vi "ExecutionView(CSM).vi"(7 "Name(\"\" to use uuid)":string="TestStandOI") -> ()   [LabVIEW 2020, in "CSMStand(Lite).lvlib"]
doc: "------------- lvcsm -------------\n[CSMStates]\nItem 0 = \"Idle\"\nItem 1 = \"CSM Documentation\"\nItem 2 = \"Error Handler\"\nItem 3 = \"VI Reference\"\nItem 4 = \"Critical Error\"\nItem 5 = \"Target Timeout Error\"\nItem 6 = \"Target Error\"\nItem 7 = \"Async Response\"\nItem 8 = \"Response\"\nItem 9 = \"Async Message Posted\"\nItem 10 = \"Initialize Core Data\"\nItem 11 = \"Exit\"\nItem 12 = \"Data: Initialize\"\nItem 13 = \"Data: Get Configuration\"\nItem 14 = \"Data: Get Internal Data\"\nItem 15 = \"Data: Set Configuration\"\nItem 16 = \"Data: Cleanup\"\nItem 17 = \"UI: Initialize\"\nItem 18 = \"UI: Cursor Set\"\nItem 19 = \"UI: Front Panel State\"\nItem 20 = \"Macro: Initialize\"\nItem 21 = \"Macro: Exit\"\nItem 22 = \"TS: Load Sequence\"\nItem 23 = \"TS: Test Started Handler\"\nItem 24 = \"TS: Step Start Handler\"\nItem 25 = \"TS: Step Complete Handler\"\nItem 26 = \"TS: Test Complete Handler\"\nItem 27 = \"Internal: action1\"\nItem 28 = \"Internal: action2\"\n\n[CSMStatus]\nItem 0 = \"Error Occurred@Error Handler\""
uses:
  CSMStand(Lite).lvlib
  <vilib>/Utility/miscctls.llb/LVRowAndColumnTypeDef.ctl
  Engine/Typedef/Def-StepComplete Event Data.ctl
  49887391-5aaa-4a15-bec5-64cc18cfe9d0.vi
  d29669de-e3bc-4aa1-abb6-bef5024a48d5.vi
  844f5a0a-3cc9-4d1a-ab8e-12611138b1fa.vi
  f99f0b71-739f-43a4-ba27-9b21da8a90fc.vi
  <userlib>/_NEVSTOP/Communicable State Machine(CSM)/_Support/Common/Format Timestamp.vi
  <userlib>/_NEVSTOP/Communicable State Machine(CSM)/AdvanceAPI/CSM - Make String Arguments Safe.vi
  <userlib>/_NEVSTOP/Communicable State Machine(CSM)/AdvanceAPI/CSM - Break Down Multiple States String.vi
  <userlib>/_NEVSTOP/Communicable State Machine(CSM)/AdvanceAPI/CSM - Compact Multiple States.vi
  <userlib>/_NEVSTOP/Communicable State Machine(CSM)/_Support/GlobalEvent/GEvt-Generate with Rule Check.vi
  <userlib>/_NEVSTOP/Communicable State Machine(CSM)/AdvanceAPI/CSM - Keywords.vi
  <userlib>/_NEVSTOP/Communicable State Machine(CSM)/_Shared/Trim Single-line Text.vi
  <userlib>/_NEVSTOP/Communicable State Machine(CSM)/_Support/GlobalEvent/Cache-GEvt Refs.vi
  <userlib>/_NEVSTOP/Communicable State Machine(CSM)/_Support/GlobalEvent/LogFilter/LogFilter - Check.vi
  <userlib>/_NEVSTOP/Communicable State Machine(CSM)/addons/API-String-Arugments-Support/_Support/Query Data as API String Arguments(variant).vi
  <userlib>/_NEVSTOP/Communicable State Machine(CSM)/addons/API-String-Arugments-Support/_Support/Convert API String Arguments to Data(variant).vi
  <userlib>/_NEVSTOP/Communicable State Machine(CSM)/_Support/GlobalEvent/LogFilter/LogFilter.lvclass
  <userlib>/_NEVSTOP/Communicable State Machine(CSM)/Communicable State Machine.lvlib
panel:
  in  "Sequence Viewer":i32(listbox)
  out "State History":string
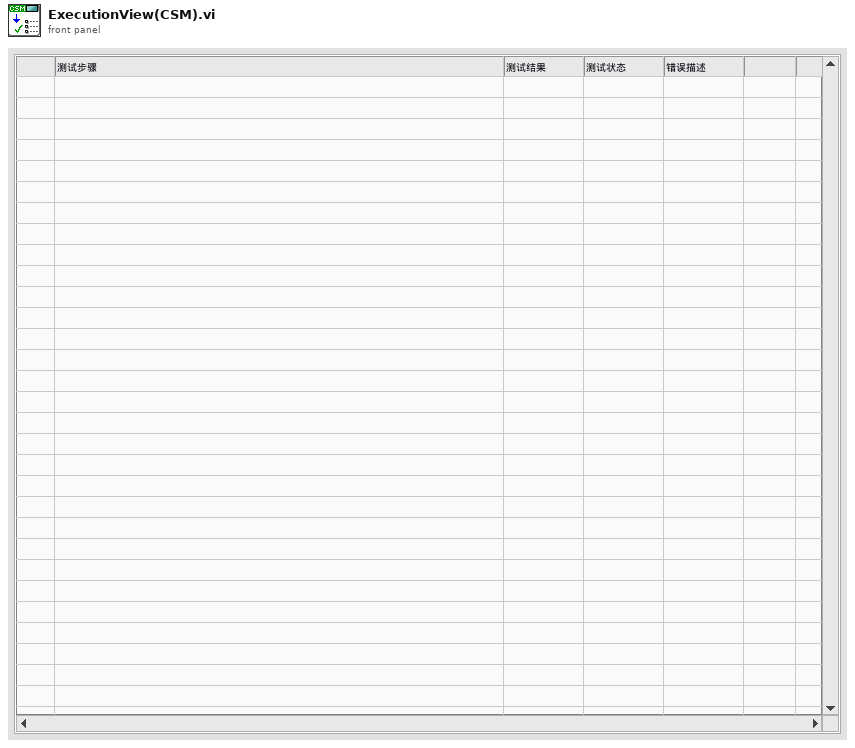
[diagram p1: front panel]
types:
  T1 = enum32{"Invalid", "Standard", "Closed", "Hidden", "Minimized", "Maximized"}
  T2 = enum32{"invalid app kind", "Development System", "Run Time System", "Student Edition", "Embedded LabVIEW", "Evaluation", "Custom"}
  T3 = typedef "LVRowAndColumnTypeDef.ctl" = cluster{"Row":i32, "Column":i32}
  T4 = typedef "CSMStand(Lite).lvlib/Def-StepComplete Event Data.ctl" = cluster{"index":i32, "Arguments":string, "error":errorcluster}
  T5 = typedef "Communicable State Machine.lvlib/_CSM_Response Source Message.ctl" = cluster{"‘State":string, "’Arguments":string, "’Error":errorcluster}
  T6 = cluster{"Current VI Reference":refnum<vi>, "Close Panel on Exit?":bool}
  T7 = cluster{"Core":cluster{"Current VI Reference":refnum<vi>, "Close Panel on Exit?":bool}, "Sequence Viewer":refnum<vi>, "ResponseMaxLen":i32}
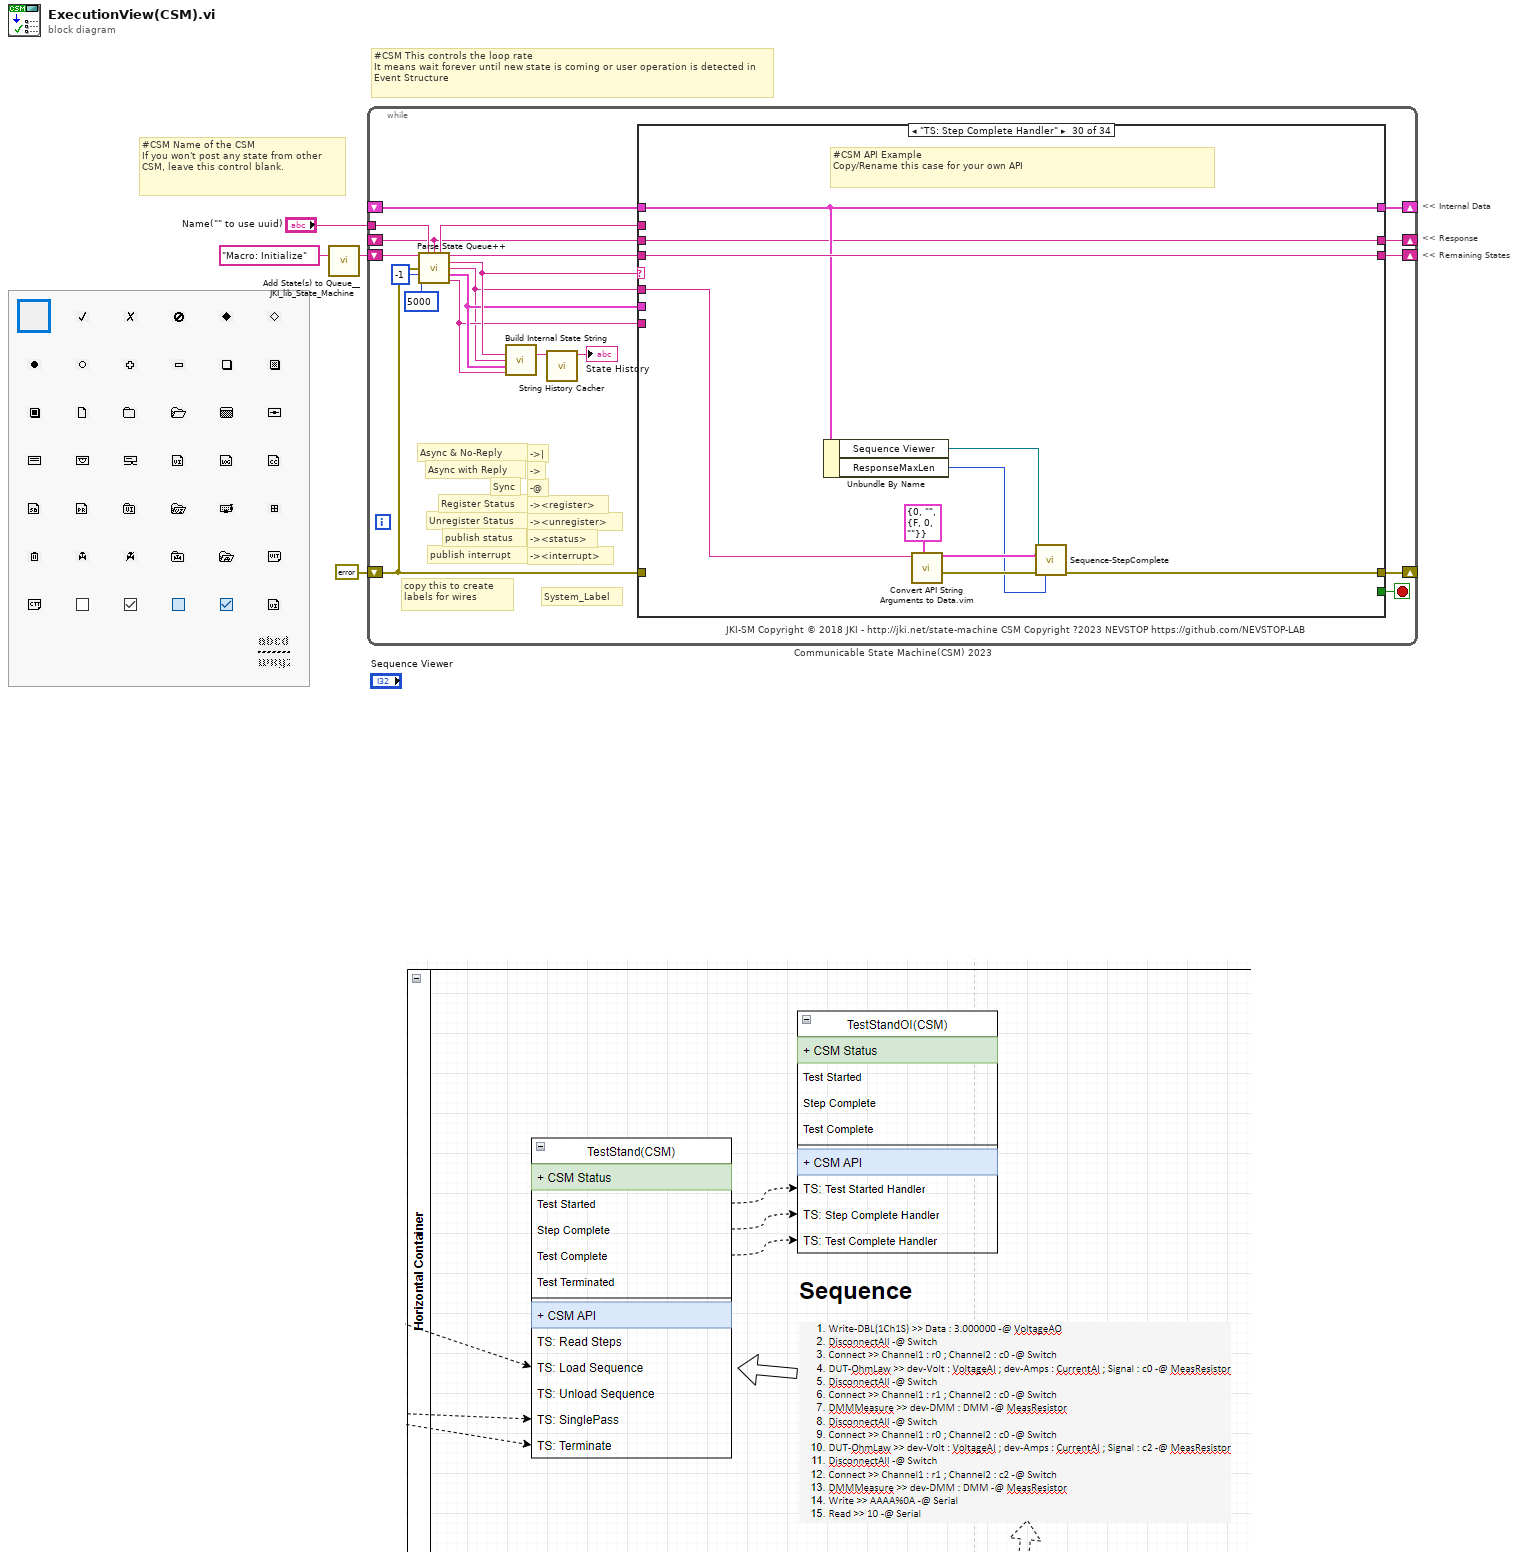
[diagram p0: block diagram]
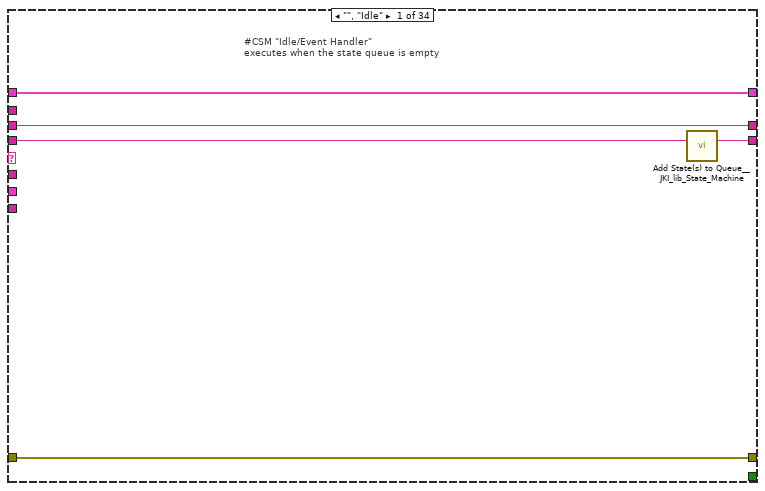
[diagram p2: hidden frame]
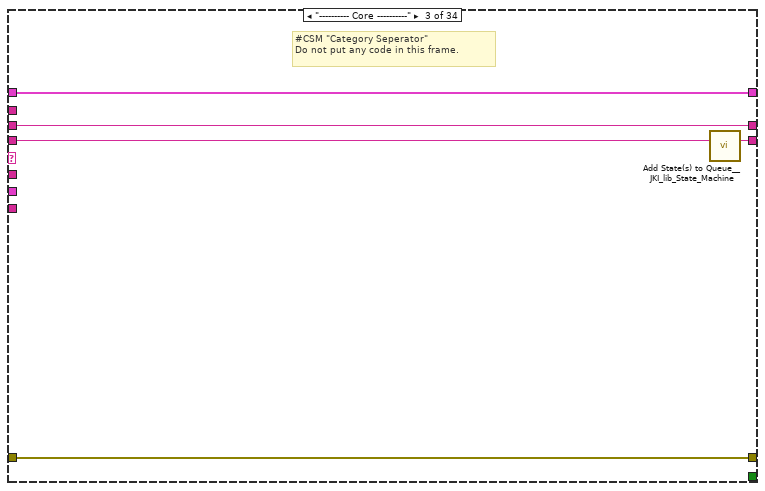
[diagram p4: hidden frame]
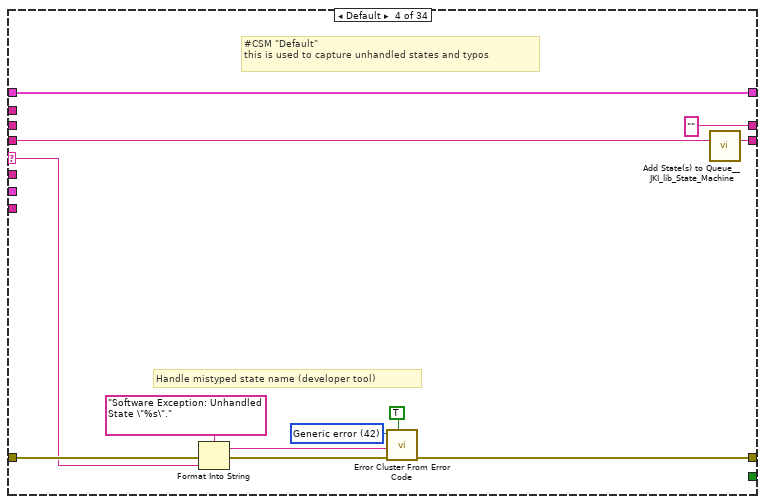
[diagram p5: hidden frame]
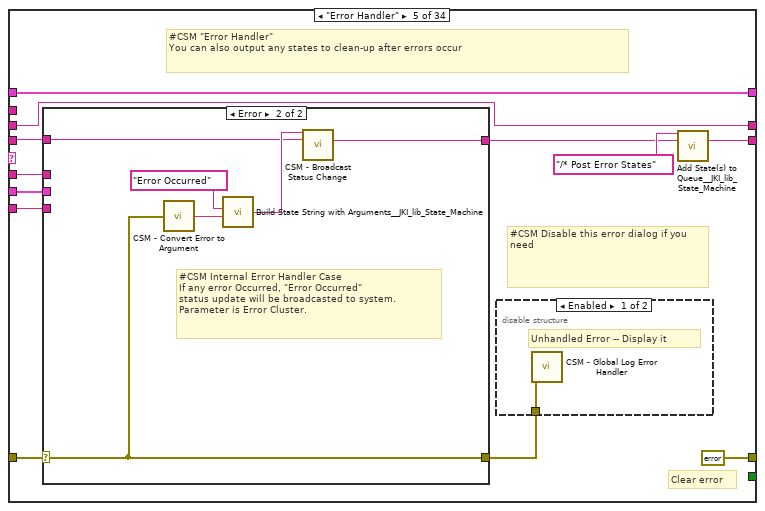
[diagram p6: hidden frame]
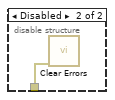
[diagram p7: hidden frame]
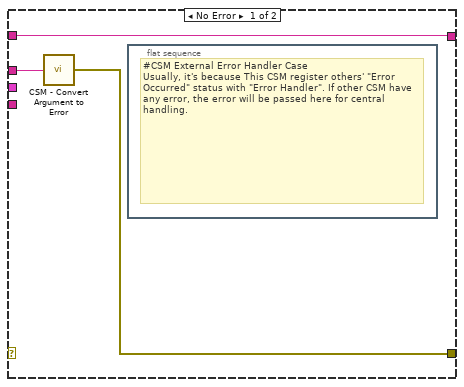
[diagram p8: hidden frame]
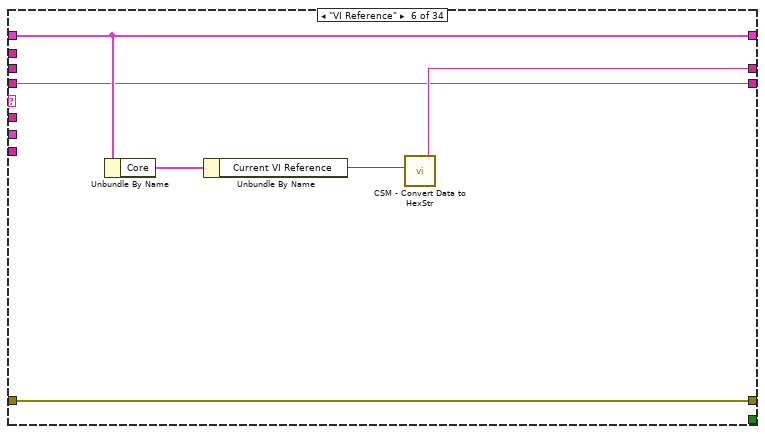
[diagram p9: hidden frame]
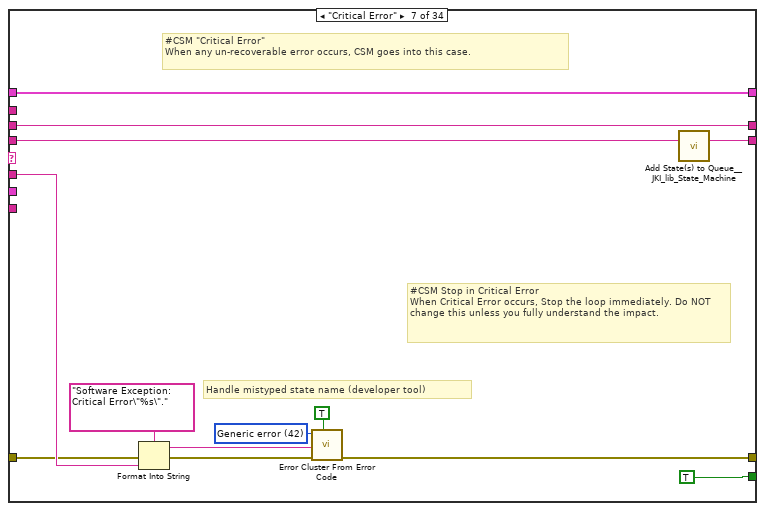
[diagram p10: hidden frame]
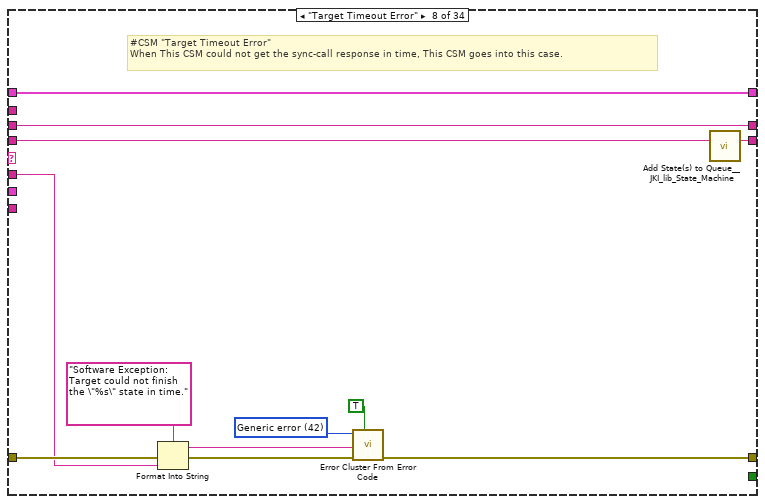
[diagram p11: hidden frame]
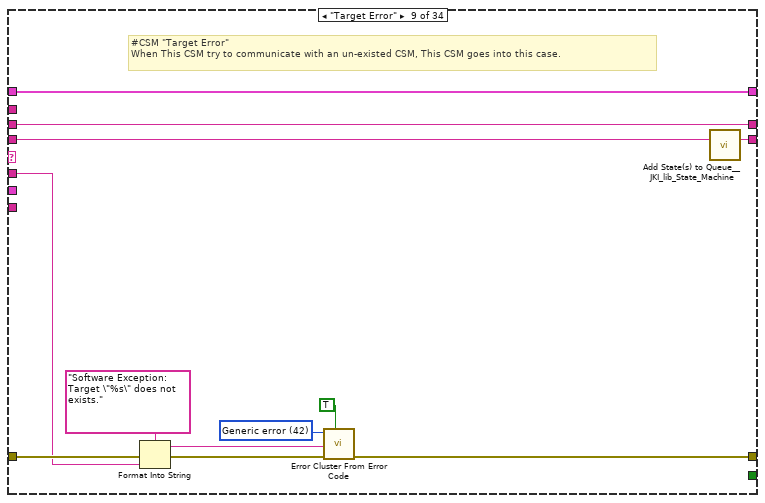
[diagram p12: hidden frame]
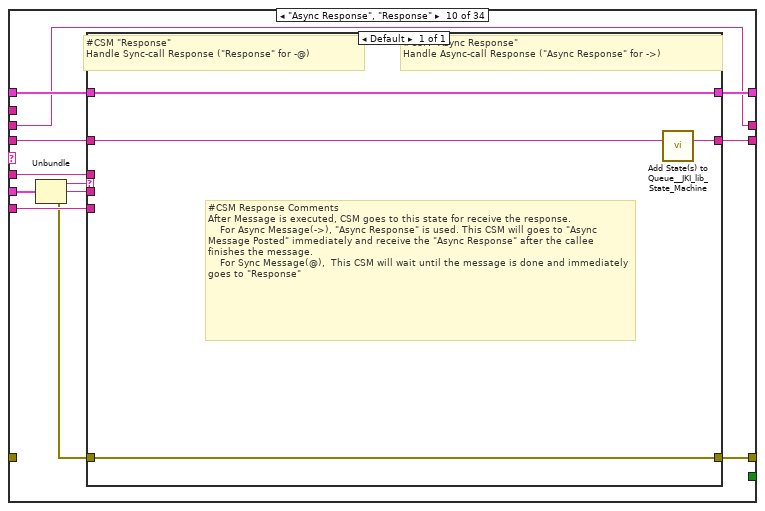
[diagram p13: hidden frame]
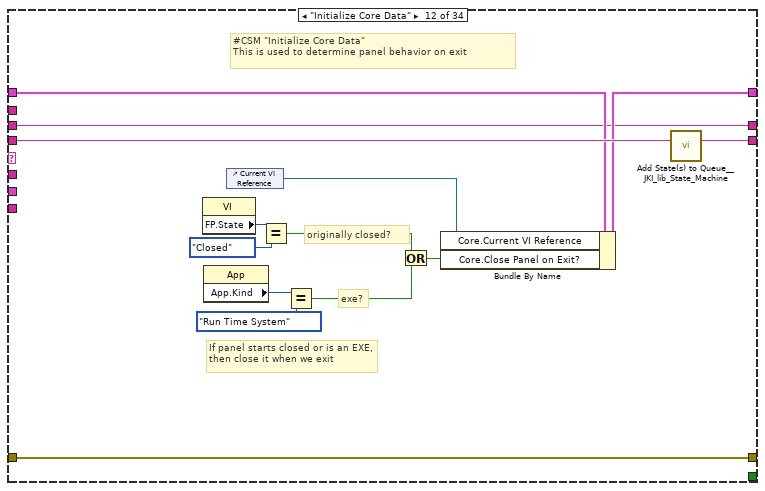
[diagram p15: hidden frame]
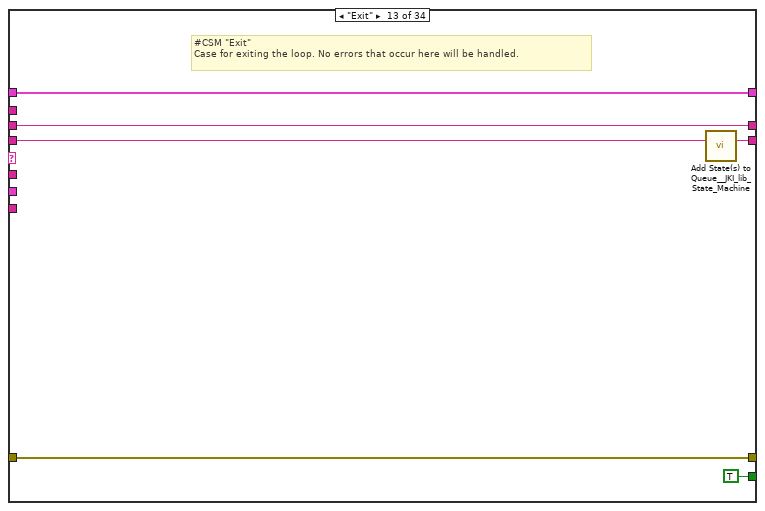
[diagram p16: hidden frame]
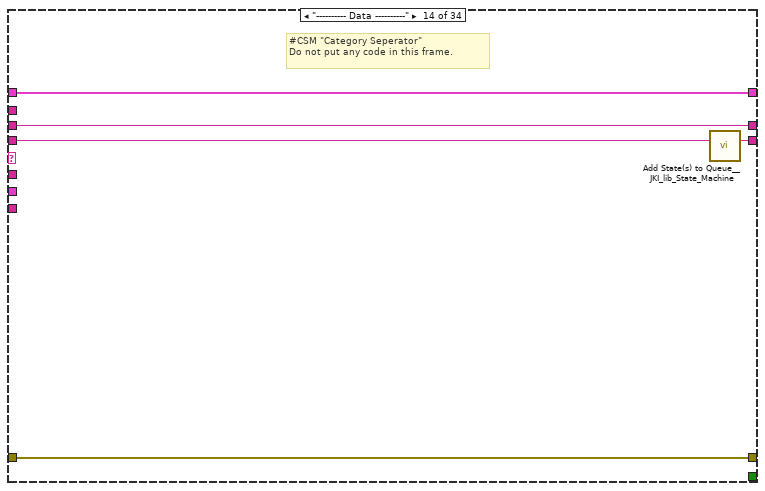
[diagram p17: hidden frame]
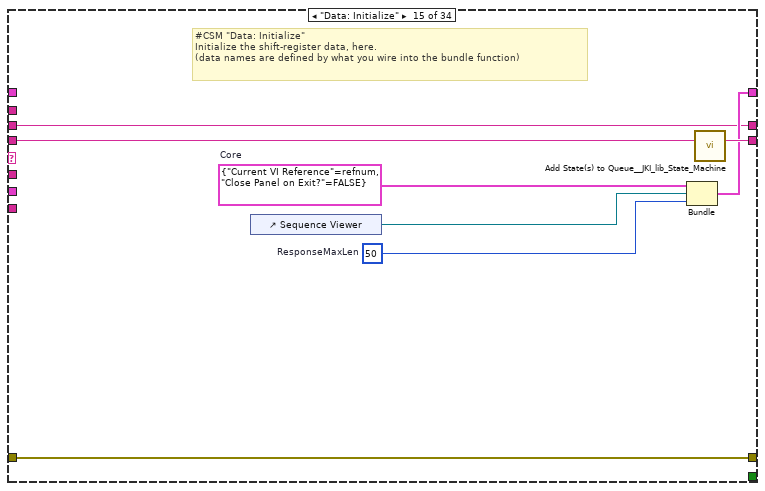
[diagram p18: hidden frame]
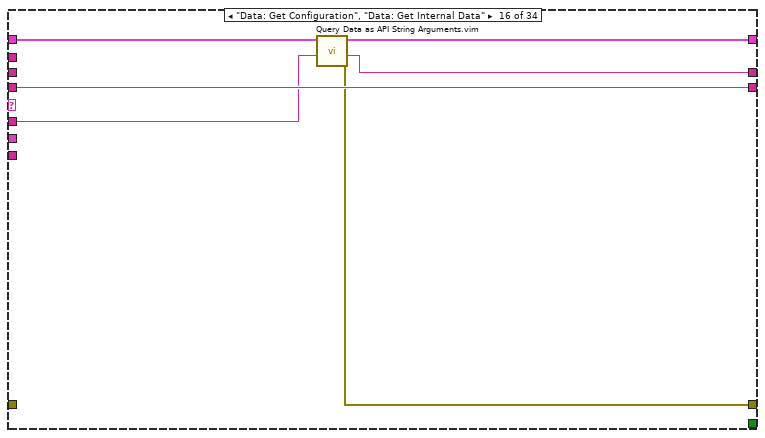
[diagram p19: hidden frame]
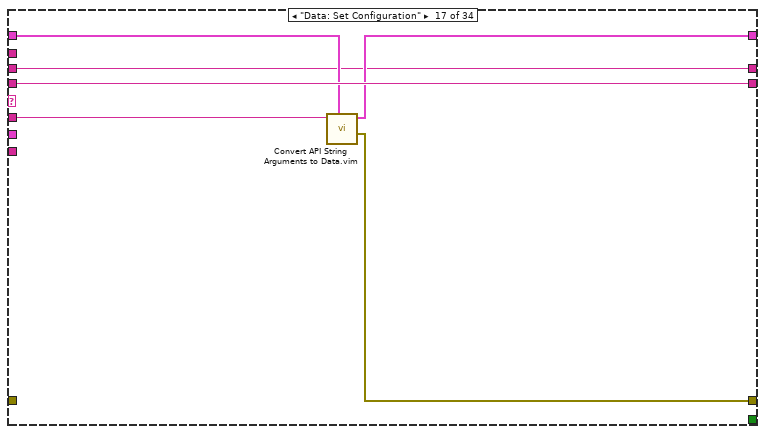
[diagram p20: hidden frame]
diagram:
  # "<< Internal Data"
  # "<< Response"
  # "<< Remaining States"
  # "#CSM Name of the CSM\nIf you won't post any state from other CSM, leave this control blank."
  # "#CSM This controls the loop rate\nIt means wait forever until new state is coming or user operation is detected in Event Structure"
  n1 = call <vilib>:"Add State(s) to Queue__JKI_lib_State_Machine.vi"("State(s) in (\"\")"="Macro: Initialize" ("Init State(\"Macro: Initialize\")")) -> ("States Out"=w1:string)  [unwired: 14 in]
  n2 = while "Communicable State Machine(CSM) 2023" {
    shift-right: [w19] -> _
    shift-left: _ -> [w18]
    shift-right: [w22] -> _
    shift-left: errorcluster {"status"=FALSE, "code"=0, "source"=""} ("error out") -> [w17]
    shift-right: [w21] -> _
    shift-left: w1 -> [w23]
    tunnel: "Name(\"\" to use uuid)" -> [w14]
    shift-right: [w15] -> _
    shift-left: _ -> [w7]
    stop <- w20 stop-if-true
    # "-><interrupt>"
    # "-><status>"
    # "-><unregister>"
    # "-><register>"
    # "-@"
    # "->"
    # "->|"
    # "publish interrupt"
    # "publish status"
    # "Unregister Status"
    # "Register Status"
    # "Sync"
    # "Async with Reply"
    # "Async & No-Reply"
    # "copy this to create labels for wires"
    # "System_Label"
    # "JKI-SM Copyright © 2018 JKI - http://jki.net/state-machine CSM Copyright ?2023 NEVSTOP https://github.com/NEVSTOP-LAB"
    n3 = call <userlib>:"Parse State Queue++.vi"("State Queue"=w23, "Name (\"\" to Use UUID)"=w14, "Response Arguments"=w7, "Previous Error"=w17, "Dequeue (1 ms)"=-1 ("Dequeue Timeout(0ms)"), "Response Timeout (-2 Use Global Settings)"=5000 ("Response Timeout(1000ms)")) -> ("Name Used"=w8:string, "Remaining States"=w24:string, "Current State"=w11:string, "Arguments"=w6:string, ">> Response Source Message >>"=w10:T5, ">> Source CSM >>"=w9:string)  [unwired: 4 in]
    n4 = call <userlib>:"Build Internal State String.vi"("State"=w11, "Arguments (\"\")"=w6, ">> Response Source Message >>"=w10, "Source (\"\")"=w9) -> ("State With Arguments"=w12:string)  [unwired: 11 in]
    n5 = call <userlib>:"String History Cacher.vi"("String"=w12) -> ("String Cache"=→"State History":string)  [unwired: 10 in]
    n6 = case shown="\"TS: Step Complete Handler\"" w11 {
      selector: w11 -> [_ _ _ w40 _ _ _ _ _ _ _ _ _ _ _ _ _ _ _ _ _ _ _ _ _ _ _ _ _ _ _ _ _ _]
      tunnel: w24 -> [w26 w33 w38 w44 w56 w75 w91 w99 w111 w127 w135 w150 w156 w161 w169 w175 w181 w188 w193 w215 w222 w238 w308 w314 w326 w329 w339 w346 w355 w365 w368 w374 w379 w384]
      tunnel: w6 -> [_ _ _ _ w54 _ w84 w95 w107 w121 _ _ _ _ _ w172 w180 _ _ _ w217 w232 _ _ _ _ w332 _ w349 w359 _ _ _ _]
      tunnel: w18 -> [w27 w32 w35 w42 w61 w79 w92 w97 w109 w125 w134 w143 w154 w158 _ w174 w179 w183 w190 w213 w220 w234 w305 w311 w323 w328 w337 w343 w354 w364 w367 w371 w376 w381]
      tunnel: [w28 w31 w36 w46 errorcluster {"status"=FALSE, "code"=0, "source"=""} ("error out") w74 w81 w94 w106 w124 w136 w147 w153 w159 w166 w170 w177 w184 w191 w197 w218 w235 w306 w312 w324 w330 w334 w341 w352 w362 w369 w372 w377 w382] -> w22
      tunnel: w17 -> [w28 w31 w36 w45 w60 w74 w82 w100 w112 _ w136 w147 w153 w159 w166 _ _ w185 w191 w210 w219 w236 w306 w312 w324 w330 w333 w344 _ _ w369 w372 w377 w382]
      tunnel: [w29 w33 w37 w43 w58 w75 w90 w98 w110 w128 w135 w149 w155 w160 w168 w175 w181 w187 w192 w214 w221 w237 w307 w313 w325 w329 w338 w345 w355 w365 w368 w373 w378 w383] -> w21
      tunnel: [_ _ _ _ _ _ TRUE _ _ _ _ _ TRUE _ _ _ _ _ _ _ _ _ _ _ _ _ _ _ _ _ _ _ _ _] -> w20
      tunnel: [w27 w32 w35 w42 w61 w79 w92 w97 w109 w126 w134 w148 w154 w158 w167 w173 w178 w183 w190 w213 w220 w234 w305 w311 w323 w328 w337 w343 w354 w364 w367 w371 w376 w381] -> w19
      tunnel: w9 -> [_ _ _ _ w53 _ _ _ _ w122 _ _ _ _ _ _ _ _ _ _ _ _ _ _ _ _ _ _ _ _ _ _ _ _]
      tunnel: w10 -> [_ _ _ _ w52 _ _ _ _ w123 _ _ _ _ _ _ _ _ _ _ _ _ _ _ _ _ _ _ _ _ _ _ _ _]
      tunnel: [w25 w30 w34 "" w51 w76 w80 w93 w105 w117 w133 w137 w151 w157 w163 w171 w176 w182 w189 w194 w216 w231 w304 w309 w315 w327 w331 w340 w347 w357 w366 w370 w375 w380] -> w15
      tunnel: w8 -> [_ _ _ _ _ _ _ _ _ _ _ _ _ _ _ _ _ _ _ _ _ _ _ _ _ _ _ _ _ _ _ _ _ _]
      tunnel: w7 -> [w25 w30 w34 _ w51 _ w80 w93 w105 w117 w133 w137 w151 w157 w163 _ w176 w182 w189 w194 w216 w231 w304 w309 w315 w327 w331 w340 w347 w357 w366 w370 w375 w380]
      frame "", "Idle" {
        # "#CSM \"Idle/Event Handler\"\nexecutes when the state queue is empty"
        n7 = call <vilib>:"Add State(s) to Queue__JKI_lib_State_Machine.vi"("State(s) in (\"\")"=w26) -> ("States Out"=w29:string)  [unwired: 14 in]
      }
      frame "CSM Documentation" {
        # "CSM Documentation"
        # "#CSM State Syntax\n\n// Comment line, all text to the right of “//” will be ignored\n// Local Message Example\nDoSth: DoA >> Arguments\n\n// Sync Call Example\nAPI: xxxx >> Arguments -@ TargetModule\n\n// Async Call Example\nAPI: xxxx >> Arguments -> TargetModule\n\n// Async Call without Reply Example\nAPI: xxxx >> Arguments ->| TargetModule\n\n// Broadcast normal status:\nStatus >> StatusArguments  -><status>\n\n// Broadcast Interrupt status:\nInterrupt >> StatusArguments  -><interrupt>\n\n// Register Source Module's status to Handler Module\nStatus@Source Module >> Handler Module@Handler Module -><register>\n\n// Unegister Source Module's status\nStatus@Source Module >> Handler Module -><unregister>"
        # "#CSM README FIRST\n\nCSM is a LabVIEW application framework that builds upon JKI State Machine (JKISM). It follows the pattern of JKISM and extends the keywords to describe message communication between CSM modules, including concepts such as Sync-Message, Async-Message, Subscription/Unsubscription of status - essential elements for creating reusable code modules. \n\nFor more information, please visit the CSM wiki: https://github.com/NEVSTOP-LAB/JKI-State-Machine-Plus-Plus/wiki\n\nFor instructions on JKI State Machine, visit: \n    http://jki.net/state-machine/\nFor information about CSM, visit: \n    https://github.com/NEVSTOP-LAB"
        # "#CSM \"Documentation\"\nCase for holding CSM Documenation"
      }
      frame "---------- Core ----------" {
        # "#CSM \"Category Seperator\"\nDo not put any code in this frame."
        n8 = call <vilib>:"Add State(s) to Queue__JKI_lib_State_Machine.vi"("State(s) in (\"\")"=w38) -> ("States Out"=w37:string)  [unwired: 14 in]
      }
      frame Default {
        w49 = 42 items=["No error", "Argument error", "Memory is full", "Out of zone", "End of file", "File already open", "Generic file I/O error", "File not found", "File permission error", "Disk is full", "Duplicate path", "Too many files open", "System feature not enabled", "Resource file not found", "Cannot add resource", "Resource not found", "Image not found", "Image memory error", "Pen does not exist", "Config type invalid", "Config token not found", "Config parse error", "Config memory error", "Bad external code format", "Bad external code offset", "External code not present", "Null window", "Destroy window error", "Null menu", "Print aborted", "Bad print record", "Print driver error", "Windows error during printing", "Memory error during printing", "Print dialog error", "Generic print error", "Invalid device refnum", "Device not found", "Device parameter error", "Device unit error", "Cannot open device", "Device call aborted", "Generic error", "Cancelled by user", "Object ID too low", "Object ID too high", "Object not in heap", "Unknown heap", "Unknown object (invalid DefProc)", "Unknown object (DefProc not in table)", "Message out of range", "Invalid (null) method", "Unknown message", "Manager call not supported", "Bad address", "Network operation in progress", "Network operation timed out", "Connection is busy", "Network attribute not supported", "Network error", "Address in use", "System out of memory", "Connection aborted", "Connection refused", "Not connected", "Already connected", "Connection closed", "Initialization error (interapplication manager)", "Bad occurrence", "Wait on unbound occurrence handler", "Occurrence queue overflow", "Datalog type conflict", "Unused", "Unrecognized type (interapplication manager)", "Memory corrupt", "Failed to make temporary DLL", "Old CIN version", "Drag socket not found", "Failed to load drop-object", "Failed to register OLE object", "Failed to release OLE object", "Format specifier type mismatch", "Unknown format specifier", "Too few format specifiers", "Too many format specifiers", "Scan failed", "Newer CIN version", "Error converting to variant", "Runtime menu error", "Password tampered", "Variant attribute not found", "Incompatible variant data type", "Event data is not available", "Event Store is not present", "Occurrence is not found", "Event Queue is not created", "Event info is not available", "Refnum passed is NULL", "Error retrieving Class GUID", "Error retrieving CoClass GUID", "Error retrieving TypeLib GUID.", "Bad built application magic bytes.", "Specific driver is different from the specific driver associated with the Logical Name.", "There is no session opened to the class driver.", "Max Error", "MAX - Error with config objects", "MAX - Error loading configuration", "MAX - Group not supported"]
        # "#CSM \"Default\"\nthis is used to capture unhandled states and typos"
        # "Handle mistyped state name (developer tool)"
        n9 = Format Into String(format string="Software Exception: Unhandled State \"%s\"." ("message"), error in=w45, w40) -> (resulting string=w48:string, error out=w47:errorcluster)  [unwired: 1 in]
        n10 = call <vilib>:"Error Cluster From Error Code.vi"("show call chain? (False)"=TRUE, "error in (no error)"=w47, "error message (\"\")"=w48, "error code (0)"=w49) -> ("error out"=w46:errorcluster)  [unwired: 5 in]
        n11 = call <vilib>:"Add State(s) to Queue__JKI_lib_State_Machine.vi"("State(s) in (\"\")"=w44) -> ("States Out"=w43:string)  [unwired: 14 in]
      }
      frame "Error Handler" {
        # "#CSM Disable this error dialog if you need"
        # "#CSM \"Error Handler\"\nYou can also output any states to clean-up after errors occur"
        # "Clear error"
        n12 = case shown="Error" w60 {
          selector: w60 -> [_ w68]
          tunnel: [w66 w70] -> w57
          tunnel: w56 -> [w66 w69]
          tunnel: [w65 w68] -> w55
          tunnel: w54 -> [w67 _]
          tunnel: w53 -> [_ _]
          tunnel: w52 -> [_ _]
          frame No Error {
            n13 = call <userlib>:"CSM - Convert Argument to Error.vi"("Argument"=w67) -> ("Error"=w65:errorcluster)  [unwired: 4 in]
            n14 = flat-sequence {
              frame #0 {
                # "#CSM External Error Handler Case\nUsually, it's because This CSM register others' \"Error Occurred\" status with \"Error Handler\". If other CSM have any error, the error will be passed here for central handling."
              }
            }
          }
          frame Error {
            # "#CSM Internal Error Handler Case \nIf any error Occurred, \"Error Occurred\" \nstatus update will be broadcasted to system.\nParameter is Error Cluster."
            n15 = call <userlib>:"CSM - Convert Error to Argument.vi"("Error"=w68) -> ("Argument"=w72:string)  [unwired: 4 in]
            n16 = call <vilib>:"Build State String with Arguments__JKI_lib_State_Machine.vi"("Arguments (\"\")"=w72, "State"="Error Occurred" ("Status with Arguments")) -> ("State with Arguments"=w71:string)  [unwired: 4 in]
            n17 = call <userlib>:"CSM - Broadcast Status Change.vi"("Status With Arguments"=w71, "State Queue"=w69) -> ("Remaining States"=w70:string)  [unwired: 13 in]
          }
        }
        n18 = disable-structure shown="Enabled" {
          disable-tunnel: w55 -> [w63 w64]
          frame Enabled {
            # "Unhandled Error -- Display it"
            n19 = call <userlib>:"CSM - Global Log Error Handler.vi"("Error In"=w63) -> ()  [unwired: 10 in, 1 out]
          }
          frame Disabled {
            n20 = call <vilib>:"Clear Errors.vi"("error in (no error)"=w64) -> ()  [unwired: 5 in, 2 out]
          }
        }
        n21 = call <vilib>:"Add State(s) to Queue__JKI_lib_State_Machine.vi"("State(s) in Front (\"\")"="/* Post Error States", "State(s) in (\"\")"=w57) -> ("States Out"=w58:string)  [unwired: 13 in]
      }
      frame "VI Reference" {
        n22 = Unbundle By Name(w79) -> ("Core"=w78:T6)
        n23 = Unbundle By Name(w78) -> ("Current VI Reference"=w77:refnum<vi>)
        n24 = call <userlib>:"CSM - Convert Data to HexStr.vi"("Variant"=w77) -> ("HEX String (0-9,A-F)"=w76:string)  [unwired: 8 in]
      }
      frame "Critical Error" {
        w88 = 42 items=["No error", "Argument error", "Memory is full", "Out of zone", "End of file", "File already open", "Generic file I/O error", "File not found", "File permission error", "Disk is full", "Duplicate path", "Too many files open", "System feature not enabled", "Resource file not found", "Cannot add resource", "Resource not found", "Image not found", "Image memory error", "Pen does not exist", "Config type invalid", "Config token not found", "Config parse error", "Config memory error", "Bad external code format", "Bad external code offset", "External code not present", "Null window", "Destroy window error", "Null menu", "Print aborted", "Bad print record", "Print driver error", "Windows error during printing", "Memory error during printing", "Print dialog error", "Generic print error", "Invalid device refnum", "Device not found", "Device parameter error", "Device unit error", "Cannot open device", "Device call aborted", "Generic error", "Cancelled by user", "Object ID too low", "Object ID too high", "Object not in heap", "Unknown heap", "Unknown object (invalid DefProc)", "Unknown object (DefProc not in table)", "Message out of range", "Invalid (null) method", "Unknown message", "Manager call not supported", "Bad address", "Network operation in progress", "Network operation timed out", "Connection is busy", "Network attribute not supported", "Network error", "Address in use", "System out of memory", "Connection aborted", "Connection refused", "Not connected", "Already connected", "Connection closed", "Initialization error (interapplication manager)", "Bad occurrence", "Wait on unbound occurrence handler", "Occurrence queue overflow", "Datalog type conflict", "Unused", "Unrecognized type (interapplication manager)", "Memory corrupt", "Failed to make temporary DLL", "Old CIN version", "Drag socket not found", "Failed to load drop-object", "Failed to register OLE object", "Failed to release OLE object", "Format specifier type mismatch", "Unknown format specifier", "Too few format specifiers", "Too many format specifiers", "Scan failed", "Newer CIN version", "Error converting to variant", "Runtime menu error", "Password tampered", "Variant attribute not found", "Incompatible variant data type", "Event data is not available", "Event Store is not present", "Occurrence is not found", "Event Queue is not created", "Event info is not available", "Refnum passed is NULL", "Error retrieving Class GUID", "Error retrieving CoClass GUID", "Error retrieving TypeLib GUID.", "Bad built application magic bytes.", "Specific driver is different from the specific driver associated with the Logical Name.", "There is no session opened to the class driver.", "Max Error", "MAX - Error with config objects", "MAX - Error loading configuration", "MAX - Group not supported"]
        # "#CSM \"Critical Error\"\nWhen any un-recoverable error occurs, CSM goes into this case."
        # "#CSM Stop in Critical Error\nWhen Critical Error occurs, Stop the loop immediately. Do NOT change this unless you fully understand the impact."
        # "Handle mistyped state name (developer tool)"
        n25 = Format Into String(format string="Software Exception: Critical Error\"%s\"." ("message"), error in=w82, w84) -> (resulting string=w87:string, error out=w86:errorcluster)  [unwired: 1 in]
        n26 = call <vilib>:"Error Cluster From Error Code.vi"("show call chain? (False)"=TRUE, "error in (no error)"=w86, "error message (\"\")"=w87, "error code (0)"=w88) -> ("error out"=w81:errorcluster)  [unwired: 5 in]
        n27 = call <vilib>:"Add State(s) to Queue__JKI_lib_State_Machine.vi"("State(s) in (\"\")"=w91) -> ("States Out"=w90:string)  [unwired: 14 in]
      }
      frame "Target Timeout Error" {
        w103 = 42 items=["No error", "Argument error", "Memory is full", "Out of zone", "End of file", "File already open", "Generic file I/O error", "File not found", "File permission error", "Disk is full", "Duplicate path", "Too many files open", "System feature not enabled", "Resource file not found", "Cannot add resource", "Resource not found", "Image not found", "Image memory error", "Pen does not exist", "Config type invalid", "Config token not found", "Config parse error", "Config memory error", "Bad external code format", "Bad external code offset", "External code not present", "Null window", "Destroy window error", "Null menu", "Print aborted", "Bad print record", "Print driver error", "Windows error during printing", "Memory error during printing", "Print dialog error", "Generic print error", "Invalid device refnum", "Device not found", "Device parameter error", "Device unit error", "Cannot open device", "Device call aborted", "Generic error", "Cancelled by user", "Object ID too low", "Object ID too high", "Object not in heap", "Unknown heap", "Unknown object (invalid DefProc)", "Unknown object (DefProc not in table)", "Message out of range", "Invalid (null) method", "Unknown message", "Manager call not supported", "Bad address", "Network operation in progress", "Network operation timed out", "Connection is busy", "Network attribute not supported", "Network error", "Address in use", "System out of memory", "Connection aborted", "Connection refused", "Not connected", "Already connected", "Connection closed", "Initialization error (interapplication manager)", "Bad occurrence", "Wait on unbound occurrence handler", "Occurrence queue overflow", "Datalog type conflict", "Unused", "Unrecognized type (interapplication manager)", "Memory corrupt", "Failed to make temporary DLL", "Old CIN version", "Drag socket not found", "Failed to load drop-object", "Failed to register OLE object", "Failed to release OLE object", "Format specifier type mismatch", "Unknown format specifier", "Too few format specifiers", "Too many format specifiers", "Scan failed", "Newer CIN version", "Error converting to variant", "Runtime menu error", "Password tampered", "Variant attribute not found", "Incompatible variant data type", "Event data is not available", "Event Store is not present", "Occurrence is not found", "Event Queue is not created", "Event info is not available", "Refnum passed is NULL", "Error retrieving Class GUID", "Error retrieving CoClass GUID", "Error retrieving TypeLib GUID.", "Bad built application magic bytes.", "Specific driver is different from the specific driver associated with the Logical Name.", "There is no session opened to the class driver.", "Max Error", "MAX - Error with config objects", "MAX - Error loading configuration", "MAX - Group not supported"]
        # "#CSM \"Target Timeout Error\"\nWhen This CSM could not get the sync-call response in time, This CSM goes into this case."
        n28 = Format Into String(format string="Software Exception: Target could not finish the \"%s\" state in time." ("message"), error in=w100, w95) -> (resulting string=w102:string, error out=w101:errorcluster)  [unwired: 1 in]
        n29 = call <vilib>:"Error Cluster From Error Code.vi"("show call chain? (False)"=TRUE, "error in (no error)"=w101, "error message (\"\")"=w102, "error code (0)"=w103) -> ("error out"=w94:errorcluster)  [unwired: 5 in]
        n30 = call <vilib>:"Add State(s) to Queue__JKI_lib_State_Machine.vi"("State(s) in (\"\")"=w99) -> ("States Out"=w98:string)  [unwired: 14 in]
      }
      frame "Target Error" {
        w115 = 42 items=["No error", "Argument error", "Memory is full", "Out of zone", "End of file", "File already open", "Generic file I/O error", "File not found", "File permission error", "Disk is full", "Duplicate path", "Too many files open", "System feature not enabled", "Resource file not found", "Cannot add resource", "Resource not found", "Image not found", "Image memory error", "Pen does not exist", "Config type invalid", "Config token not found", "Config parse error", "Config memory error", "Bad external code format", "Bad external code offset", "External code not present", "Null window", "Destroy window error", "Null menu", "Print aborted", "Bad print record", "Print driver error", "Windows error during printing", "Memory error during printing", "Print dialog error", "Generic print error", "Invalid device refnum", "Device not found", "Device parameter error", "Device unit error", "Cannot open device", "Device call aborted", "Generic error", "Cancelled by user", "Object ID too low", "Object ID too high", "Object not in heap", "Unknown heap", "Unknown object (invalid DefProc)", "Unknown object (DefProc not in table)", "Message out of range", "Invalid (null) method", "Unknown message", "Manager call not supported", "Bad address", "Network operation in progress", "Network operation timed out", "Connection is busy", "Network attribute not supported", "Network error", "Address in use", "System out of memory", "Connection aborted", "Connection refused", "Not connected", "Already connected", "Connection closed", "Initialization error (interapplication manager)", "Bad occurrence", "Wait on unbound occurrence handler", "Occurrence queue overflow", "Datalog type conflict", "Unused", "Unrecognized type (interapplication manager)", "Memory corrupt", "Failed to make temporary DLL", "Old CIN version", "Drag socket not found", "Failed to load drop-object", "Failed to register OLE object", "Failed to release OLE object", "Format specifier type mismatch", "Unknown format specifier", "Too few format specifiers", "Too many format specifiers", "Scan failed", "Newer CIN version", "Error converting to variant", "Runtime menu error", "Password tampered", "Variant attribute not found", "Incompatible variant data type", "Event data is not available", "Event Store is not present", "Occurrence is not found", "Event Queue is not created", "Event info is not available", "Refnum passed is NULL", "Error retrieving Class GUID", "Error retrieving CoClass GUID", "Error retrieving TypeLib GUID.", "Bad built application magic bytes.", "Specific driver is different from the specific driver associated with the Logical Name.", "There is no session opened to the class driver.", "Max Error", "MAX - Error with config objects", "MAX - Error loading configuration", "MAX - Group not supported"]
        # "#CSM \"Target Error\"\nWhen This CSM try to communicate with an un-existed CSM, This CSM goes into this case."
        n31 = Format Into String(format string="Software Exception: Target \"%s\" does not exists." ("message"), error in=w112, w107) -> (resulting string=w114:string, error out=w113:errorcluster)  [unwired: 1 in]
        n32 = call <vilib>:"Error Cluster From Error Code.vi"("show call chain? (False)"=TRUE, "error in (no error)"=w113, "error message (\"\")"=w114, "error code (0)"=w115) -> ("error out"=w106:errorcluster)  [unwired: 5 in]
        n33 = call <vilib>:"Add State(s) to Queue__JKI_lib_State_Machine.vi"("State(s) in (\"\")"=w111) -> ("States Out"=w110:string)  [unwired: 14 in]
      }
      frame "Async Response", "Response" {
        # "#CSM \"Async Response\"\nHandle Async-call Response (\"Async Response\" for ->)"
        # "#CSM \"Response\"\nHandle Sync-call Response (\"Response\" for -@)"
        n34 = Unbundle(w123) -> ("‘State"=w120:string, "’Arguments"=w119:string, "’Error"=w118:errorcluster)
        n35 = case shown="Default" w120 {
          tunnel: [w129] -> w128
          tunnel: w127 -> [w130]
          tunnel: [w132] -> w126
          tunnel: w125 -> [w132]
          tunnel: [w131] -> w124
          tunnel: w118 -> [w131]
          tunnel: w122 -> [_]
          tunnel: w121 -> [_]
          tunnel: w119 -> [_]
          frame Default {
            # "#CSM Response Comments\nAfter Message is executed, CSM goes to this state for receive the response.\n    For Async Message(->), \"Async Response\" is used. This CSM will goes to \"Async Message Posted\" immediately and receive the \"Async Response\" after the callee finishes the message.\n    For Sync Message(@),  This CSM will wait until the message is done and immediately goes to \"Response\""
            n36 = call <vilib>:"Add State(s) to Queue__JKI_lib_State_Machine.vi"("State(s) in (\"\")"=w130) -> ("States Out"=w129:string)  [unwired: 14 in]
          }
        }
      }
      frame "Async Message Posted" {
        # "#CSM \"Async Message Posted\"\nAfter Async Message is posted (-> or ->| ), CSM goes to this state for post-action.\nYou can use Argument - State to tell which Async Message is called."
      }
      frame "Initialize Core Data" {
        # "#CSM \"Initialize Core Data\"\nThis is used to determine panel behavior on exit"
        # "originally closed?"
        # "exe?"
        # "If panel starts closed or is an EXE, then close it when we exit"
        n37 = property class="VI"() -> ("FP.State"=w140:T1)  [unwired: 2 in, 2 out]
        n38 = property class="App"() -> ("App.Kind"=w146:T2)  [unwired: 2 in, 2 out]
        n39 = control-ref of="Current VI Reference"() -> (w141:refnum<vi>)
        n40 = Equal?(x=w140, y=T1."Closed" ("Front Panel Window:State")) -> (x = y?=w138:bool)
        n41 = Equal?(x=w146, y=T2."Run Time System" ("Application:Kind")) -> (x = y?=w144:bool)
        n42 = Or(x=w138, y=w144) -> (x .or. y?=w142:bool)
        n43 = Bundle By Name(cluster=w143, "Core.Current VI Reference"=w141, "Core.Close Panel on Exit?"=w142) -> (w148:T7)
        n44 = call <vilib>:"Add State(s) to Queue__JKI_lib_State_Machine.vi"("State(s) in (\"\")"=w150) -> ("States Out"=w149:string)  [unwired: 14 in]
      }
      frame "Exit" {
        # "#CSM \"Exit\"\nCase for exiting the loop. No errors that occur here will be handled."
        n45 = call <vilib>:"Add State(s) to Queue__JKI_lib_State_Machine.vi"("State(s) in (\"\")"=w156) -> ("States Out"=w155:string)  [unwired: 14 in]
      }
      frame "---------- Data ----------" {
        # "#CSM \"Category Seperator\"\nDo not put any code in this frame."
        n46 = call <vilib>:"Add State(s) to Queue__JKI_lib_State_Machine.vi"("State(s) in (\"\")"=w161) -> ("States Out"=w160:string)  [unwired: 14 in]
      }
      frame "Data: Initialize" {
        w162 = 50  # ResponseMaxLen
        w165 = T6 {"Current VI Reference"=refnum, "Close Panel on Exit?"=FALSE}  # Core
        # "#CSM \"Data: Initialize\"\nInitialize the shift-register data, here.\n(data names are defined by what you wire into the bundle function)"
        n47 = control-ref of="Sequence Viewer"() -> (w164:refnum<vi>)
        n48 = Bundle("Core"=w165, "Sequence Viewer"=w164, "ResponseMaxLen"=w162) -> (w167:T7)  [unwired: 1 in]
        n49 = call <vilib>:"Add State(s) to Queue__JKI_lib_State_Machine.vi"("State(s) in (\"\")"=w169) -> ("States Out"=w168:string)  [unwired: 14 in]
      }
      frame "Data: Get Configuration", "Data: Get Internal Data" {
        n50 = call "Query Data as API String Arguments.vim"("Setting Name"=w172, "Internal Data"=w174) -> ("error"=w170:errorcluster, "Setting as String"=w171:string, "Internal Data(dup)"=w173:T7)  [unwired: 7 in]
      }
      frame "Data: Set Configuration" {
        n51 = call "Convert API String Arguments to Data.vim"("Type"=w179, "String"=w180) -> ("error"=w177:errorcluster, "Data"=w178:T7)  [unwired: 6 in]
      }
      frame "Data: Cleanup" {
        # "#CSM \"Data: Cleanup\"\nCleanup any data and references, here.\n(this is called automatically, by the Macro: Exit)"
        n52 = Unbundle By Name(w183) -> ("Core.Current VI Reference"=w186:refnum<vi>)
        n53 = Close Reference(reference=w186, error in (no error)=w185) -> (error out=w184:errorcluster)
        n54 = call <vilib>:"Add State(s) to Queue__JKI_lib_State_Machine.vi"("State(s) in (\"\")"=w188) -> ("States Out"=w187:string)  [unwired: 14 in]
      }
      frame "---------- UI ----------" {
        # "#CSM \"Category Seperator\"\nDo not put any code in this frame."
        n55 = call <vilib>:"Add State(s) to Queue__JKI_lib_State_Machine.vi"("State(s) in (\"\")"=w193) -> ("States Out"=w192:string)  [unwired: 14 in]
      }
      frame "UI: Initialize" {
        # "#CSM \"UI: Initialize\"\nInitialize the User Interface, here.\n(this is called automatically, by the Macro: Init)"
        n56 = Unbundle By Name(w213) -> ("Sequence Viewer"=w212:refnum<vi>)
        n57 = property class="MCListbox (strict)"(reference=w212, error in=w210, "ItemNames"=string[][] [] ("Item Names"), "Vertical Lines Visible"=TRUE ("Visible Items:Vertical Lines Visible"), "Horizontal Lines Visible"=TRUE ("Visible Items:Horizontal Lines Visible"), "Symbols Vis"=TRUE ("Visible Items:Symbols Visible"), "ColHdrString"=string[] ["", "测试步骤", "测试结果", "测试状态", "错误描述"] ("Column Header Strings[]"), "ActiveCell"=T3 {"Row"=-1, "Column"=-2} ("Active Cell:Active Cell"), "Justify"=enum16{"Left", "Center", "Right"}."Center" ("Active Cell:Cell Justification")) -> (reference out=w201:refnum<vi>, error out=w200:errorcluster)
        n58 = property class="MCListbox (strict)"(reference=w201, error in=w200, "ActiveCell"=T3 {"Row"=-2, "Column"=-2} ("Active Cell:Active Cell"), "CellBG"=u32 16448250) -> (reference out=w199:refnum<vi>, error out=w198:errorcluster)
        n59 = property class="MCListbox (strict)"(reference=w199, error in=w198, "ActiveCell"=T3 {"Row"=-1, "Column"=-2} ("Active Cell:Active Cell"), "CellBG"=u32 15263976) -> (error out=w197:errorcluster)  [unwired: 1 out]
        n60 = call <vilib>:"Add State(s) to Queue__JKI_lib_State_Machine.vi"("State(s) in (\"\")"=w215) -> ("States Out"=w214:string)  [unwired: 14 in]
      }
      frame "UI: Cursor Set" {
        # "Argument"
        # "#CSM \"UI: Cursor Set\"\nSet and Unset Cursor Busy.\n(Usage: \"UI: Cursor Set >> Busy|Idle\")"
        n61 = disable-structure shown="Default" {
          disable-tunnel: w219 -> [w225 w230]
          disable-tunnel: [w224 w230] -> w218
          disable-tunnel: w217 -> [w223 _]
          frame condition #0 (active) {
            n62 = case shown="\"Busy\"" w223 {
              tunnel: w225 -> [w227 w229]
              tunnel: [w226 w228] -> w224
              frame "Idle", Default {
                n63 = call <vilib>:"Unset Busy.vi"("error in (no error)"=w227) -> ("error out"=w226:errorcluster)  [unwired: 10 in]
              }
              frame "Busy" {
                n64 = call <vilib>:"Set Busy.vi"("error in (no error)"=w229) -> ("error out"=w228:errorcluster)  [unwired: 9 in, 1 out]
              }
            }
          }
          frame condition #1 {
          }
        }
        n65 = call <vilib>:"Add State(s) to Queue__JKI_lib_State_Machine.vi"("State(s) in (\"\")"=w222) -> ("States Out"=w221:string)  [unwired: 14 in]
      }
      frame "UI: Front Panel State" {
        # "Argument"
        # "#CSM \"UI: Front Panel State\"\nSet Front Panel Open or Closed\n(Usage: \"UI: Front Panel State >> Open|Close\")"
        n66 = Unbundle By Name(w234) -> ("Core.Current VI Reference"=w233:refnum<vi>)
        n67 = case shown="\"Minimize\", \"Minimized\"" w232 {
          tunnel: w236 -> [w244 w259 w270 w283 w296]
          tunnel: [w246 w260 w272 w285 w298] -> w235
          tunnel: w233 -> [w245 w257 w271 w284 w297]
          frame "Open", "Standard", Default {
            w239 = T1."Standard" ("State")
            n68 = property class="VI"(reference=w245, error in=w244) -> (reference out=w242:refnum<vi>, error out=w243:errorcluster, "FP.State"=w241:T1)
            n69 = Not Equal?(x=w241, y=w239) -> (x != y?=w240:bool)
            n70 = case shown="True" w240 {
              tunnel: [w250 w252] -> w246
              tunnel: w243 -> [w249 w252]
              tunnel: w242 -> [w248 _]
              tunnel: w239 -> [w247 _]
              frame True {
                n71 = invoke class="VI" method="FP.Open"(reference=w248, error in=w249, "Activate"=TRUE, "State"=w247) -> (error out=w250:errorcluster)  [unwired: 1 in, 4 out]
              }
              frame False {
              }
            }
          }
          frame "Close", "Closed" {
            n72 = property class="VI"(reference=w257, error in=w259) -> (reference out=w256:refnum<vi>, error out=w258:errorcluster, "FP.State"=w254:T1)
            n73 = Not Equal?(x=w254, y=T1."Closed" ("Front Panel Window:State")) -> (x != y?=w253:bool)
            n74 = case shown="True" w253 {
              tunnel: [w261 w264] -> w260
              tunnel: w258 -> [w261 w263]
              tunnel: w256 -> [_ w262]
              frame False {
              }
              frame True {
                n75 = invoke class="VI" method="FP.Close"(reference=w262, error in=w263) -> (error out=w264:errorcluster)  [unwired: 1 in, 2 out]
              }
            }
          }
          frame "Hidden", "Hide" {
            w265 = T1."Hidden" ("State")
            n76 = property class="VI"(reference=w271, error in=w270) -> (reference out=w268:refnum<vi>, error out=w269:errorcluster, "FP.State"=w267:T1)
            n77 = Not Equal?(x=w267, y=w265) -> (x != y?=w266:bool)
            n78 = case shown="True" w266 {
              tunnel: [w276 w277] -> w272
              tunnel: w269 -> [w275 w277]
              tunnel: w268 -> [w274 _]
              tunnel: w265 -> [w273 _]
              frame True {
                n79 = invoke class="VI" method="FP.Open"(reference=w274, error in=w275, "State"=w273) -> (error out=w276:errorcluster)  [unwired: 2 in, 4 out]
              }
              frame False {
              }
            }
          }
          frame "Minimize", "Minimized" {
            w278 = T1."Minimized" ("State")
            n80 = property class="VI"(reference=w284, error in=w283) -> (reference out=w281:refnum<vi>, error out=w282:errorcluster, "FP.State"=w280:T1)
            n81 = Not Equal?(x=w280, y=w278) -> (x != y?=w279:bool)
            n82 = case shown="False" w279 {
              tunnel: [w289 w290] -> w285
              tunnel: w282 -> [w288 w290]
              tunnel: w281 -> [w287 _]
              tunnel: w278 -> [w286 _]
              frame True {
                n83 = invoke class="VI" method="FP.Open"(reference=w287, error in=w288, "State"=w286) -> (error out=w289:errorcluster)  [unwired: 2 in, 4 out]
              }
              frame False {
              }
            }
          }
          frame "Maximize", "Maximized" {
            w291 = T1."Maximized" ("State")
            n84 = property class="VI"(reference=w297, error in=w296) -> (reference out=w294:refnum<vi>, error out=w295:errorcluster, "FP.State"=w293:T1)
            n85 = Not Equal?(x=w293, y=w291) -> (x != y?=w292:bool)
            n86 = case shown="True" w292 {
              tunnel: [w302 w303] -> w298
              tunnel: w295 -> [w301 w303]
              tunnel: w294 -> [w300 _]
              tunnel: w291 -> [w299 _]
              frame True {
                n87 = invoke class="VI" method="FP.Open"(reference=w300, error in=w301, "State"=w299) -> (error out=w302:errorcluster)  [unwired: 2 in, 4 out]
              }
              frame False {
              }
            }
          }
        }
        n88 = call <vilib>:"Add State(s) to Queue__JKI_lib_State_Machine.vi"("State(s) in (\"\")"=w238) -> ("States Out"=w237:string)  [unwired: 14 in]
      }
      frame "---------- Macro ----------" {
        # "#CSM \"Category Seperator\"\nDo not put any code in this frame."
        n89 = call <vilib>:"Add State(s) to Queue__JKI_lib_State_Machine.vi"("State(s) in (\"\")"=w308) -> ("States Out"=w307:string)  [unwired: 14 in]
      }
      frame "Macro: Initialize" {
        w310 = "Data: Initialize\nInitialize Core Data\n//Events: Register\nUI: Initialize\n//UI: Front Panel State >> Open"  # Data: Initialize Initialize Core Data //Events: Register UI: Initialize //UI: Front Panel State >> Open
        # "#CSM \"Macro: Initialize\"\nInitialization Macro (This is called once, when the VI starts)"
        n90 = call <vilib>:"Add State(s) to Queue__JKI_lib_State_Machine.vi"("State(s) in Front (\"\")"=w310, "State(s) in (\"\")"=w314) -> ("States Out"=w313:string)  [unwired: 13 in]
      }
      frame "Macro: Exit" {
        # "#CSM \"Macro: Exit\"\nExit Macro (This is called once, when the VI exits)"
        n91 = Unbundle By Name(w323) -> ("Core.Close Panel on Exit?"=w322:bool)
        n92 = Select(t="UI: Front Panel State >> Close", s=w322, f="") -> (s? t:f=w319:string)
        n93 = call <vilib>:"Add State(s) to Queue__JKI_lib_State_Machine.vi"("State(s) in Front (\"\")"="//Exit Sub-Modules ", "State(s) in (\"\")"=w319, "State(s) at Back (\"\")"="Data: Cleanup\n//Events: Unregister\nExit") -> ("States Out"=w317:string)  [unwired: 12 in]
        n94 = call <vilib>:"Add State(s) to Queue__JKI_lib_State_Machine.vi"("State(s) in Front (\"\")"=w317, "State(s) in (\"\")"=w326) -> ("States Out"=w325:string)  [unwired: 13 in]
      }
      frame "---------- API ----------" {
        # "#CSM \"Category Seperator\"\nDo not put any code in this frame."
      }
      frame "TS: Load Sequence" {
        # "#CSM API Example\nCopy/Rename this case for your own API"
        n95 = Unbundle By Name(w337) -> ("Sequence Viewer"=w336:refnum<vi>)
        n96 = call <userlib>:"CSM - Revert Arguments-Safe String.vi"("Safe Argument String"=w332) -> ("Origin Argument String"=w335:string)  [unwired: 8 in]
        n97 = call "Sequence-Load.vi"("error in (no error)"=w333, "Sequence String"=w335, "MCListbox Refnum"=w336) -> ("error out"=w334:errorcluster)  [unwired: 7 in, 1 out]
        n98 = call <vilib>:"Add State(s) to Queue__JKI_lib_State_Machine.vi"("State(s) in (\"\")"=w339) -> ("States Out"=w338:string)  [unwired: 14 in]
      }
      frame "TS: Test Started Handler" {
        # "#CSM API Example\nCopy/Rename this case for your own API"
        n99 = Unbundle By Name(w343) -> ("Sequence Viewer"=w342:refnum<vi>)
        n100 = call "Sequence-Started.vi"("error in (no error)"=w344, "MCListbox Refnum"=w342) -> ("error out"=w341:errorcluster)  [unwired: 8 in, 1 out]
        n101 = call <vilib>:"Add State(s) to Queue__JKI_lib_State_Machine.vi"("State(s) in (\"\")"=w346) -> ("States Out"=w345:string)  [unwired: 14 in]
      }
      frame "TS: Step Start Handler" {
        # "#CSM API Example\nCopy/Rename this case for your own API"
        n102 = call "Convert API String Arguments to Data.vim"("Type"=T4 {"index"=0, "Arguments"="", "error"={"status"=FALSE, "code"=0, "source"=""}} ("StepComplete Event Data"), "String"=w349) -> ("error"=w350:errorcluster, "Data"=w348:T4)  [unwired: 6 in]
        n103 = Unbundle By Name(w354) -> ("Sequence Viewer"=w353:refnum<vi>)
        n104 = call "Sequence-StepStart.vi"("MCListbox Refnum"=w353, "Step Feedback"=w348, "error in (no error)"=w350) -> ("error out"=w352:errorcluster)  [unwired: 11 in, 1 out]
      }
      frame "TS: Step Complete Handler" {
        # "#CSM API Example\nCopy/Rename this case for your own API"
        n105 = Unbundle By Name(w364) -> ("Sequence Viewer"=w363:refnum<vi>, "ResponseMaxLen"=w356:i32)
        n106 = call "Convert API String Arguments to Data.vim"("Type"=T4 {"index"=0, "Arguments"="", "error"={"status"=FALSE, "code"=0, "source"=""}} ("StepComplete Event Data"), "String"=w359) -> ("error"=w360:errorcluster, "Data"=w358:T4)  [unwired: 6 in]
        n107 = call "Sequence-StepComplete.vi"("MCListbox Refnum"=w363, "Step Feedback"=w358, "error in (no error)"=w360, "length (rest)"=w356) -> ("error out"=w362:errorcluster)  [unwired: 10 in, 1 out]
      }
      frame "TS: Test Complete Handler" {
        # "#CSM API Example\nCopy/Rename this case for your own API"
      }
      frame "---------- Internal ----------" {
        # "#CSM \"Category Seperator\"\nDo not put any code in this frame."
        n108 = call <vilib>:"Add State(s) to Queue__JKI_lib_State_Machine.vi"("State(s) in (\"\")"=w374) -> ("States Out"=w373:string)  [unwired: 14 in]
      }
      frame "Internal: action1" {
        # "#CSM \"Internal State\"\nThis category is used for holding internal states"
        n109 = call <vilib>:"Add State(s) to Queue__JKI_lib_State_Machine.vi"("State(s) in (\"\")"=w379) -> ("States Out"=w378:string)  [unwired: 14 in]
      }
      frame "Internal: action2" {
        # "#CSM \"Internal State\"\nThis category is used for holding internal states"
        n110 = call <vilib>:"Add State(s) to Queue__JKI_lib_State_Machine.vi"("State(s) in (\"\")"=w384) -> ("States Out"=w383:string)  [unwired: 14 in]
      }
    }
  }
